vi "Close.vi"(8 "error in (no error)":errorcluster, 11 "reference in":refnum<class "DUT_Handler_Base.lvclass">) -> (0 "error out":errorcluster, 3 "reference in":refnum<class "DUT_Handler_Base.lvclass">)   [LabVIEW 2022 SP3, in "DUT_Handler_Base.lvlib" / "DUT_Handler_Base.lvclass"]
uses:
  DUT_Handler_Base.lvclass
  Components/ViPER.lvlibp/ViPER.lvclass
  C:/Projects/Medulla/ViPER/Examples/Flux_Capacitor_Tester/Components/ViPER.lvlibp/ViPER.lvclass
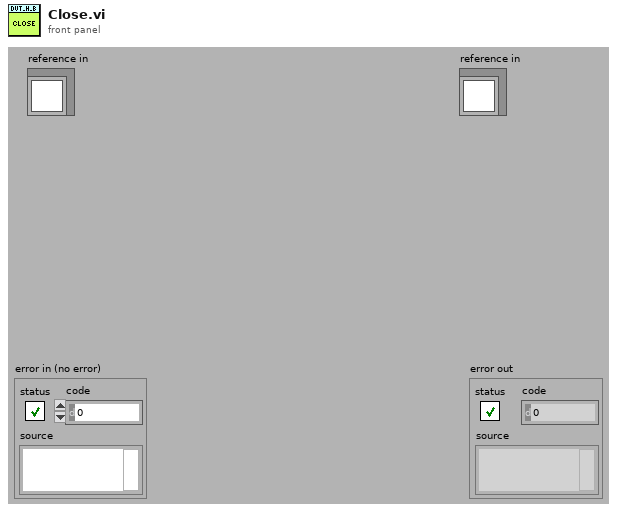
[diagram p1: front panel]
types:
  T1 = typedef "DUT_Handler_Base.lvlib/DUT_Handler_Base.lvclass/ObjectAttributes.ctl" = cluster{"Config":T2, "Event":refnum<user-event>}
  T2 = typedef "DUT_Handler_Base.lvlib/DUT_Handler_Base.lvclass/Config.ctl" = cluster{"default":string}
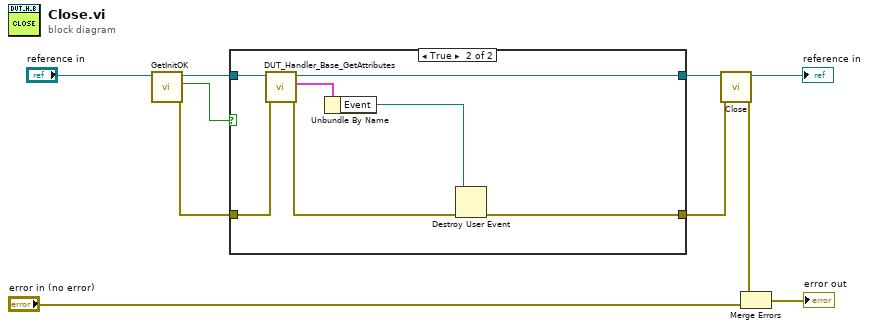
[diagram p0: block diagram]
diagram:
  n1 = call "GetInitOK.vi"("reference in"="reference in") -> ("error out"=w4:errorcluster, "init_ok"=w5:bool, "reference out"=w6:refnum<class "DUT_Handler_Base.lvclass">)  [unwired: 8 in]
  n2 = case shown="True" w5 {
    tunnel: w4 -> [w12 w18]
    tunnel: [w12 w13] -> w7
    tunnel: w6 -> [w11 w19]
    tunnel: [w11 w16] -> w8
    frame False {
    }
    frame True {
      n3 = call "DUT_Handler_Base_GetAttributes.vi"("error in (no error)"=w18, "reference in"=w19) -> ("error out"=w14:errorcluster, "Data"=w17:T1, "reference out"=w16:refnum<class "DUT_Handler_Base.lvclass">)  [unwired: 6 in, 1 out]
      n4 = Unbundle By Name(w17) -> ("Event"=w15:refnum<user-event>)
      n5 = Destroy User Event(user event=w15, error in=w14) -> (error out=w13:errorcluster)
    }
  }
  n6 = call-parent "Close.vi"("error in (no error)"=w7, "reference in"=w8) -> ("error out"=w3:errorcluster, "reference out"=→"reference in":refnum<class "DUT_Handler_Base.lvclass">)  [unwired: 8 in]
  n7 = Merge Errors(w3, "error in (no error)") -> (→"error out":errorcluster)
